vi "Init Matrix.vi"(8 "error in (no error)":errorcluster, 11 "Grove 2 RGB LED Matrix in":refnum<class "Grove 2 RGB LED Matrix.lvclass">) -> (0 "error out":errorcluster, 2 "Version":string, 3 "Grove 2 RGB LED Matrix out":refnum<class "Grove 2 RGB LED Matrix.lvclass">)   [LabVIEW 2020, in "CTI-Peripheral.lvlib" / "Grove 2 RGB LED Matrix.lvclass"]
uses:
  Grove 2 RGB LED Matrix.lvclass
  Data Types/MatrixI2CCommand.ctl
  Grove 2 RGB LED Matrix.lvclass/Grove 2 RGB LED Matrix.ctl
  CTI/I2C Connection/I2C Connection.lvclass/I2C Connection.ctl
  CTI/Session/I2C Write Data.vi
  CTI/Session/I2C Read Data.vi
  CTI/I2C Connection/I2C Connection.lvclass
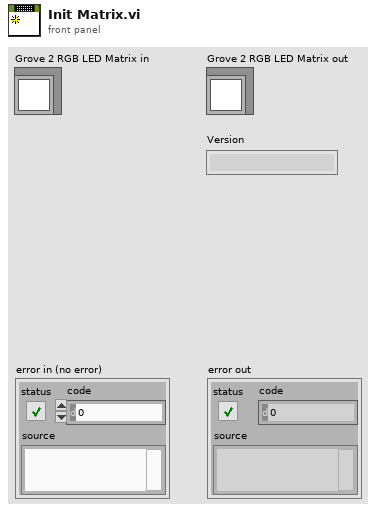
[diagram p1: front panel]
types:
  T1 = typedef "CTI-Peripheral.lvlib/Grove 2 RGB LED Matrix.lvclass/MatrixI2CCommand.ctl" = u8
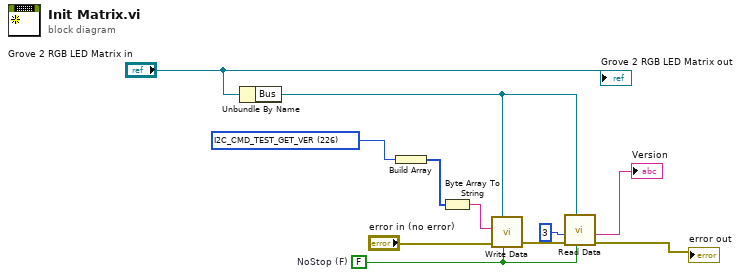
[diagram p0: block diagram]
diagram:
  w2 = T1 226 items=["I2C_CMD_GET_DEV_ID"=0, "I2C_CMD_DISP_BAR"=1, "I2C_CMD_DISP_EMOJI"=2, "I2C_CMD_DISP_NUM"=3, "I2C_CMD_DISP_STR"=4, "I2C_CMD_DISP_CUSTOM"=5, "I2C_CMD_DISP_OFF"=6, "I2C_CMD_DISP_ASCII"=7, "I2C_CMD_DISP_FLASH"=8, "I2C_CMD_DISP_COLOR_BAR"=9, "I2C_CMD_DISP_COLOR_WAVE"=10, "I2C_CMD_DISP_COLOR_CLOCKWISE"=11, "I2C_CMD_DISP_COLOR_ANIMATION"=12, "I2C_CMD_DISP_COLOR_BLOCK "=13, "I2C_CMD_CONTINUE_DATA"=129, "I2C_CMD_STORE_FLASH"=160, "I2C_CMD_DELETE_FLASH"=161, "I2C_CMD_LED_ON"=176, "I2C_CMD_LED_OFF"=177, "I2C_CMD_AUTO_SLEEP_ON"=178, "I2C_CMD_AUTO_SLEEP_OFF"=179, "I2C_CMD_DISP_ROTATE"=180, "I2C_CMD_DISP_OFFSET"=181, "I2C_CMD_SET_ADDR"=192, "I2C_CMD_RST_ADDR"=193, "I2C_CMD_TEST_GET_VER"=226, "I2C_CMD_GET_DEVICE_UID"=241] ("I2C Command")
  w10 = FALSE  # NoStop (F)
  n1 = Unbundle By Name("Grove 2 RGB LED Matrix in") -> ("Bus"=w5:refnum<class "I2C Connection.lvclass">)
  n2 = Build Array(w2) -> (w1:T1[])
  n3 = Byte Array To String(unsigned byte array=w1) -> (string=w8:string)
  n4 = call "Write Data.vi"("NoStop (F)"=w10, "I2C Connection"=w5, "error in (no error)"="error in (no error)", "Data"=w8) -> ("error out"=w9:errorcluster)  [unwired: 7 in]
  n5 = call "Read Data.vi"("NoStop (F)"=w10, "I2C Connection"=w5, "error in (no error)"=w9, "Len"=u8 3 ("Read Len")) -> ("error out"=→"error out":errorcluster, "Data"=→"Version":string)  [unwired: 6 in]
  "Grove 2 RGB LED Matrix out" <- "Grove 2 RGB LED Matrix in"
